vi "controlTargetRange.vi"(7 "Set":bool, 8 "error in":errorcluster, 9 "Target Range [nm/µdeg]":i32, 10 "axis in":u8, 11 "connection ID":refnum<k5>) -> (0 "error out":errorcluster, 1 "Target Range [nm/µdeg] out":i32, 2 "axis out":u8, 3 "connection ID":refnum<k5>)   [LabVIEW 2016, in "AMC_VIs.lvlib"]
doc: "This function retrieves or sets the range around the target position in which the flag \"In Target Range\" (see VIII.7.a) becomes active."
uses:
  AMC_VIs.lvlib
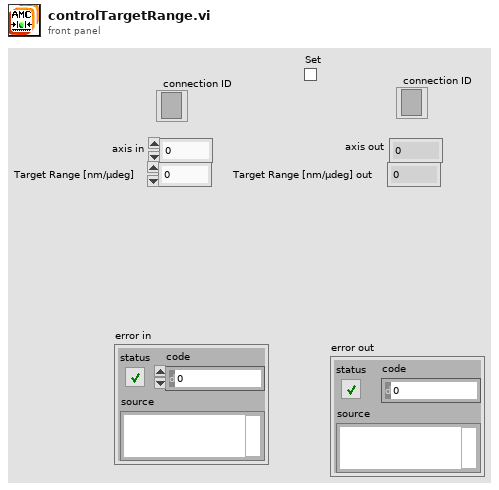
[diagram p1: front panel]
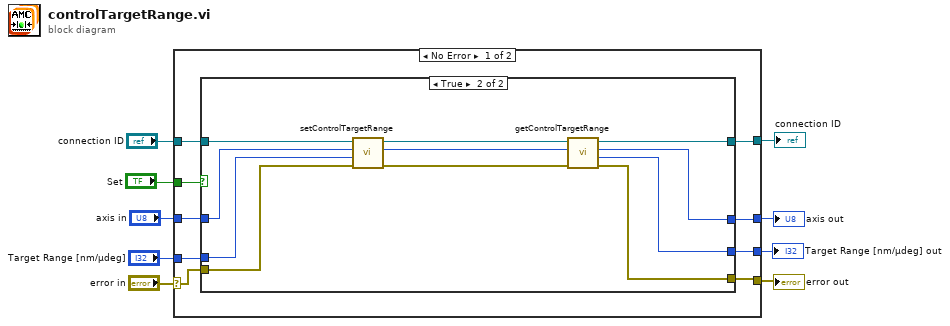
[diagram p0: block diagram]
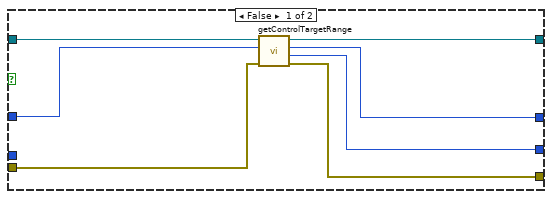
[diagram p2: hidden frame]
diagram:
  n1 = case shown="No Error" "error in" {
    selector: "error in" -> [w10 w40]
    tunnel: "axis in" -> [w16 w38]
    tunnel: [w11 w40] -> w8
    tunnel: [w13 w38] -> w7
    tunnel: "Target Range [nm/µdeg]" -> [w15 w39]
    tunnel: [w12 w39] -> w5
    tunnel: "Set" -> [w17 _]
    tunnel: [w14 w37] -> w3
    tunnel: "connection ID" -> [w18 w37]
    frame No Error {
      n2 = case shown="True" w17 {
        tunnel: [w24 w31] -> w14
        tunnel: w18 -> [w25 w36]
        tunnel: w16 -> [w23 w35]
        tunnel: [w19 w28] -> w13
        tunnel: [w21 w26] -> w11
        tunnel: [w20 w27] -> w12
        tunnel: w15 -> [_ w33]
        tunnel: w10 -> [w22 w34]
        frame False {
          n3 = call "getControlTargetRange.vi"("error in"=w22, "axis"=w23, "connection ID"=w25) -> ("error out"=w21:errorcluster, "targetrange"=w20:i32, "axis_out"=w19:i32, "connection ID"=w24:refnum<k5>)  [unwired: 5 in]
        }
        frame True {
          n4 = call "setControlTargetRange.vi"("error in"=w34, "range"=w33, "axis"=w35, "connection ID"=w36) -> ("error out"=w29:errorcluster, "axis_out"=w30:i32, "connection ID"=w32:refnum<k5>)  [unwired: 5 in]
          n5 = call "getControlTargetRange.vi"("error in"=w29, "axis"=w30, "connection ID"=w32) -> ("error out"=w26:errorcluster, "targetrange"=w27:i32, "axis_out"=w28:i32, "connection ID"=w31:refnum<k5>)  [unwired: 5 in]
        }
      }
    }
    frame Error {
    }
  }
  "error out" <- w8
  "axis out" <- w7
  "Target Range [nm/µdeg] out" <- w5
  "connection ID" <- w3
